vi "L_SAVE_DATA_Set.vi"(6 "数值 4":i32, 9 "数值 5":i32, 10 "数值 3":i32, 11 "board PF":bool[](array[boolean])) -> (1 "数值":i32, 2 "数组":string[](array[string]), 3 "字符串":string, 4 "数值 2":i32)   [LabVIEW 2018]
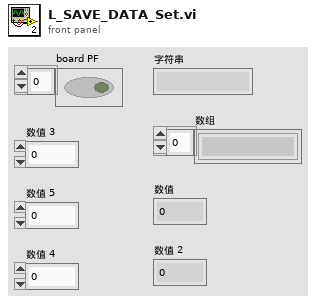
[diagram p1: front panel]
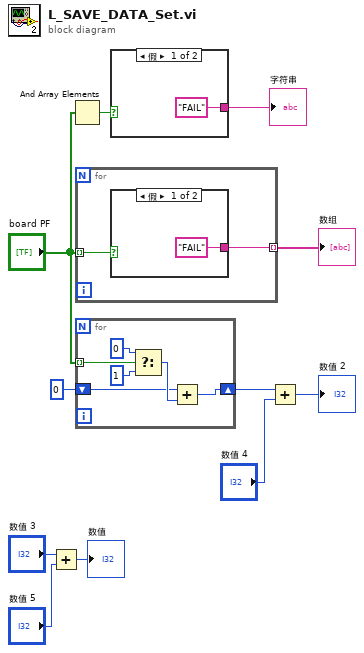
[diagram p0: block diagram]
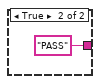
[diagram p2: hidden frame]
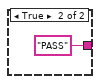
[diagram p3: hidden frame]
diagram:
  n1 = Add(x="数值 3", y="数值 5") -> (x+y=→"数值":i32)
  n2 = And Array Elements(Boolean array="board PF") -> (logical AND=w1:bool)
  n3 = for {
    tunnel: "board PF" -> [w13] mode=indexing
    tunnel: [w12] -> w4 mode=indexing
    n4 = case shown="假" w13 {
      tunnel: ["FAIL" "PASS" ("字符串")] -> w12
      frame False {
      }
      frame True {
      }
    }
  }
  "数组" <- w4
  n5 = for {
    shift-right: [w16] -> w5
    shift-left: i16 0 -> [w17]
    tunnel: "board PF" -> [w18] mode=indexing
    n6 = Select(t=i16 0 ("精度(6)"), s=w18, f=i16 1 ("精度(6)")) -> (s? t:f=w19:i16)
    n7 = Add(x=w17, y=w19) -> (x+y=w16:i16)
  }
  n8 = case shown="假" w1 {
    tunnel: ["FAIL" "PASS" ("字符串")] -> w10
    frame False {
    }
    frame True {
    }
  }
  "字符串" <- w10
  n9 = Add(x=w5, y="数值 4") -> (x+y=→"数值 2":i32)
